vi "Create Async Mask.vi"(8 "error in (no error)":errorcluster, 11 "Parameter In":T1 {"Base Word" format="%04d"; "Address" format="%04x"; "Mask" format="%04x"; "Value" format="%016x"}) -> (0 "error out":errorcluster, 3 "Parameter Out":T1 {"Base Word" format="%04d"; "Address" format="%04x"; "Mask" format="%04x"; "Value" format="%016x"})   [LabVIEW 2020, in "BCI-1553 API.lvlib" / "Async Message.lvclass"]
doc: "Prepares the mask for the data that needs to be read/written for this asynchronous Message."
uses:
  Async Message.lvclass
  TypeDefs/Parameter Table Data.ctl
  TypeDefs/Scaling Information.ctl
  BCI-1553 API.lvlib
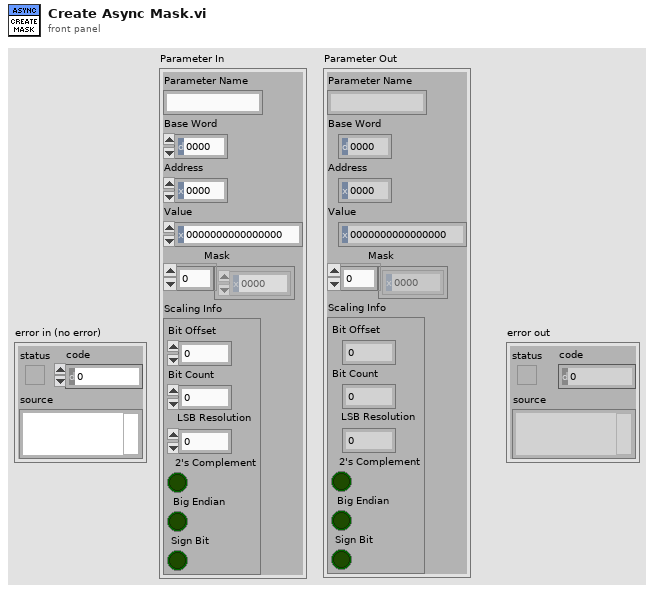
[diagram p1: front panel]
types:
  T1 = typedef "BCI-1553 API.lvlib/Parameter Table Data.ctl" = cluster{"Parameter Name":string, "Base Word":u16, "Address":u16, "Value":u64, "Mask":u16[], "Scaling Info":T2}
  T2 = typedef "BCI-1553 API.lvlib/Scaling Information.ctl" = cluster{"Bit Offset":i32, "Bit Count":i32, "LSB Resolution":dbl, "2's Complement":bool, "Big Endian":bool, "Sign Bit":bool}
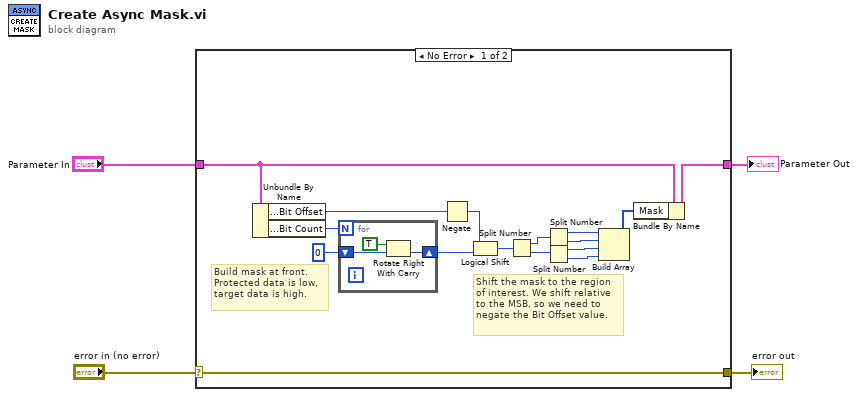
[diagram p0: block diagram]
diagram:
  n1 = case shown="No Error" "error in (no error)" {
    selector: "error in (no error)" -> [w20 w24]
    tunnel: [w20 w24] -> w3
    tunnel: "Parameter In" -> [w6 _]
    tunnel: [w5 _] -> w1
    frame No Error {
      # "Shift the mask to the region\nof interest. We shift relative\nto the MSB, so we need to\nnegate the Bit Offset value."
      # "Build mask at front.\nProtected data is low,\ntarget data is high."
      n2 = Unbundle By Name(w6) -> ("Scaling Info.Bit Offset"=w8:i32, "Scaling Info.Bit Count"=w19:i32)
      n3 = for {
        N: w19 -> [_]
        shift-right: [w22] -> w17
        shift-left: u64 0 -> [w23]
        n4 = Rotate Right With Carry(2:w23, 3:TRUE ("carry")) -> (0:w22:u64)  [unwired: 1 out]
      }
      n5 = Negate(x=w8) -> (-x=w7:i32)
      n6 = Logical Shift(y=w7, x=w17) -> (x << y=w10:u64)
      n7 = Split Number(x=w10) -> (hi(x)=w11:u32, lo(x)=w16:u32)
      n8 = Split Number(x=w11) -> (hi(x)=w15:u16, lo(x)=w14:u16)
      n9 = Split Number(x=w16) -> (hi(x)=w13:u16, lo(x)=w12:u16)
      n10 = Build Array(w15, w14, w13, w12) -> (w9:u16[])
      n11 = Bundle By Name(cluster=w6, "Mask"=w9) -> (w5:T1)
    }
    frame Error {
    }
  }
  "error out" <- w3
  "Parameter Out" <- w1
